vi "niFPGA Rational Resampler Template.vi"(0 "input data":fxp<+/-,16,1>) -> (3 "channel index":u8, 4 "output data":fxp<+/-,18,1> format="%.18g", 10 "output valid":bool)   [LabVIEW 2017]
doc: "Integer Resampler"
uses:
  <vilib>/Platform/TimedLoop/XDataNode/timing_clust.ctl
  <vilib>/Platform/TimedLoop/XDataNode/nitl_modes.ctl
  <vilib>/Platform/TimedLoop/XDataNode/wakeup.ctl
  <vilib>/Platform/TimedLoop/XDataNode/XDataNode.xnode
  <vilib>/Platform/TimedLoop/XDataNode/XDNodeRunTimeDep.lvlib
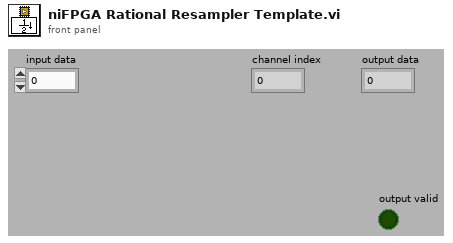
[diagram p1: front panel]
types:
  T1 = typedef "XDNodeRunTimeDep.lvlib/timing_clust.ctl" = cluster{"Expected End [f-1]":u64, "Actual End [f-1]":u64, "Finished Late? [f-1]":bool, "Expected End [i-1]":u64, "Actual End [i-1]":u64, "Finished Late? [i-1]":bool, "Expected Start [i]":u64, "Actual Start [i]":u64, "Expected Start [f]":u64, "Actual Start [f]":u64, "Source Name":string, "Structure Name":string, "Period":i64, "Deadline":i64, "Offset":i64, "Start":i64, "Priority":i32, "Timeout":i32, "Mode":T2, "Wakeup Reason":T3, "Error":errorcluster, "Source Type":string, "Secondary Source Type":string, "Global End Time":u64, "Global Start Time":u64, "Frame Duration":u64, "Iteration Duration":u64, "Assigned CPU":i32, "I/O Scan Engine Mode":u32}
  T2 = typedef "XDNodeRunTimeDep.lvlib/nitl_modes.ctl" = enum32{"No Change", "Process missed periods, maintain original phase", "Discard missed periods, maintain original phase", "Process missed periods, ignore original phase", "Discard missed periods, ignore original phase"}
  T3 = typedef "XDNodeRunTimeDep.lvlib/wakeup.ctl" = enum32{"Normal", "Aborted", "Asynchronous wakeup", "Timing source error", "Timed loop error", "Timeout"}
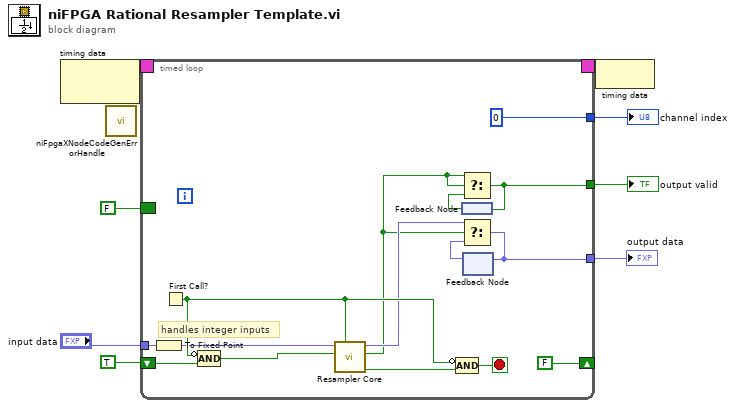
[diagram p0: block diagram]
diagram:
  n1 = node-c288 ("Input Node")() -> (w8:T1)  [unwired: 1 out]
  n2 = call <vilib>:"niFpgaXNodeCodeGenErrorHandle.vi"() -> ()  [unwired: 1 in]
  n3 = timed-loop "Timed Loop" {
    timing: w8 -> [_]
    timing-out: [_] -> w7
    tunnel: "input data" -> [w10]
    tunnel: [w18] -> w2
    tunnel: [w20] -> w3
    border: FALSE ("dataReady?") -> [_]
    tunnel: [u8 0] -> w4
    shift-right: [FALSE] -> _
    shift-left: TRUE -> [w21]
    stop <- w19 stop-if-true
    # "handles integer inputs"
    n4 = To Fixed-Point(number=w10) -> (fixed-point=w9:fxp<+/-,16,1>)  [unwired: 1 in]
    n5 = First Call?() -> (First Call?: T/F=w14:bool)
    n6 = Compound Arithmetic op=AND(invert w14, w21) -> (w15:bool)
    n7 = call "Resampler Core"("reset"=w14, "dataRDYIn"=w15, "datain"=w9) -> ("idle?"=w11:bool, "dataReadyOut"=w12:bool, "output data"=w13:fxp<+/-,18,1>)  [unwired: 6 in]
    n8 = Compound Arithmetic op=AND(invert w14, w11) -> (w19:bool)
    n9 = feedback #1() -> (w23:bool)
    n10 = Select(t=w12, s=w12, f=w23) -> (s? t:f=w20:bool)
    n11 = feedback-in #1(w20) -> ()
    n12 = feedback #2() -> (w17:fxp<+/-,18,1>)  [unwired: 1 out]
    n13 = Select(t=w13, s=w12, f=w17) -> (s? t:f=w18:fxp<+/-,18,1>)
    n14 = feedback-in #2(w18) -> ()
  }
  "channel index" <- w4
  "output valid" <- w3
  "output data" <- w2
  n15 = node-c288 ("Output Node")(w7) -> ()
